vi "Write Bit Field.vi"(5 "occurrence":refnum<k4>, 6 "IL Echo(true)":bool=TRUE, 7 "Close IL Connections (T)":bool=TRUE, 8 "error in (no error)":errorcluster, 9 "Interlock Chain":refnum<class "Interlock Chain.lvclass">, 10 "Bit Field":u16, 11 "Valve in":refnum<class "Valve.lvclass">) -> (0 "error out":errorcluster, 1 "Interlock occured?":bool, 3 "Valve out":refnum<class "Valve.lvclass">)   [LabVIEW 2015, in "cRIO-Carbondioxide.lvlib" / "CO2-Actor.lvlib" / "Valve.lvclass"]
uses:
  Valve.lvclass
  Interlocks/Interlock Chain/Interlock Chain.lvclass
  <vilib>/ActorFramework/Actor/Actor.lvclass/Actor.ctl
  <vilib>/ActorFramework/Message Enqueuer/Message Enqueuer.lvclass/Message Enqueuer.ctl
  Valve.lvclass/Valve.ctl
  <vilib>/ActorFramework/Actor/Read Self Enqueuer.vi
  <vilib>/ActorFramework/Message Enqueuer/Init from Existing Queue.vi
  <vilib>/ActorFramework/Message Enqueuer/Message Enqueuer.lvclass
  <vilib>/ActorFramework/Actor/Actor.lvclass
  CO2 Actor/CO2 Actor.lvclass
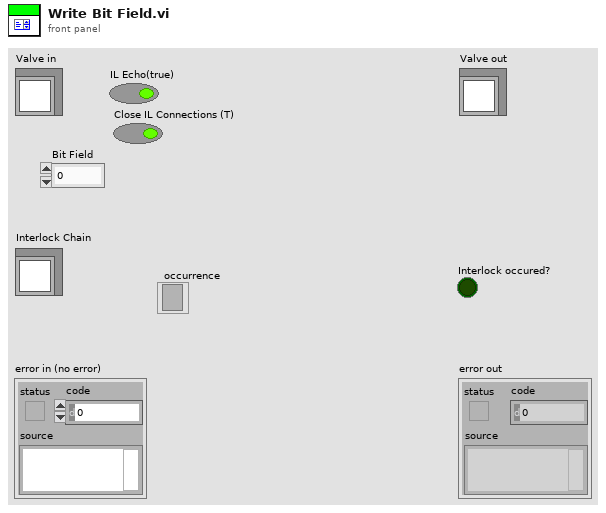
[diagram p1: front panel]
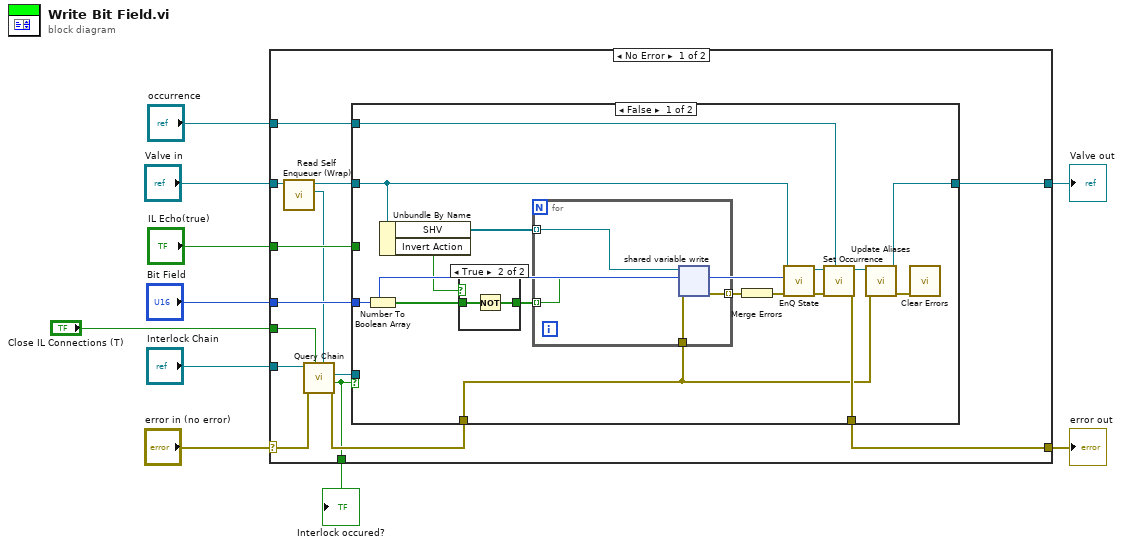
[diagram p0: block diagram]
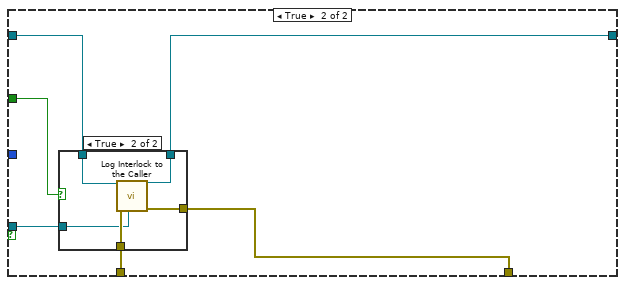
[diagram p3: hidden frame]
diagram:
  n1 = case shown="No Error" "error in (no error)" {
    selector: "error in (no error)" -> [w21 w62]
    tunnel: [w23 w62] -> w9
    tunnel: [w24 w61] -> w7
    tunnel: "Valve in" -> [w13 w61]
    tunnel: "Interlock Chain" -> [w22 _]
    tunnel: "Bit Field" -> [w19 _]
    tunnel: "IL Echo(true)" -> [w17 _]
    tunnel: "Close IL Connections (T)" -> [w16 _]
    tunnel: [w15 _] -> w2
    tunnel: "occurrence" -> [w14 _]
    frame No Error {
      n2 = call "Read Self Enqueuer (Wrap).vi"("CO2 Actor in"=w13) -> ("Actor Framework:Message Enqueuer"=w11:refnum<class "Message Enqueuer.lvclass">, "CO2 Actor out"=w12:refnum<class "Valve.lvclass">)  [unwired: 9 in]
      n3 = call "Query Chain.vi"("Caller Enqueuer"=w11, "Close Connections (F)"=w16, "error in (no error)"=w21, "Interlock Chain"=w22) -> ("error out"=w20:errorcluster, "Interlock?"=w15:bool, "Interlock out"=w18:refnum<class "Interlock.lvclass">)  [unwired: 2 in, 3 out]
      n4 = case shown="False" w15 {
        tunnel: [w34 w50] -> w24
        tunnel: w12 -> [w36 w53]
        tunnel: [w28 w49] -> w23
        tunnel: w20 -> [w25 w52]
        tunnel: w19 -> [w35 _]
        tunnel: w18 -> [_ w51]
        tunnel: w17 -> [_ w48]
        tunnel: w14 -> [w26 _]
        frame False {
          n5 = Number To Boolean Array(number=w35) -> (Boolean array=w39:bool[])
          n6 = Unbundle By Name(w36) -> ("SHV"=w40:refnum<k21>[], "Invert Action"=w31:bool)
          n7 = case shown="True" w31 {
            tunnel: w39 -> [w41 w43]
            tunnel: [w41 w42] -> w32
            frame False {
            }
            frame True {
              n8 = Not(x=w43) -> (.not. x?=w42:bool[])
            }
          }
          n9 = for {
            tunnel: w40 -> [w47] mode=indexing
            tunnel: w32 -> [w45] mode=indexing
            tunnel: w25 -> [w46]
            tunnel: [w44] -> w38 mode=indexing
            n10 = shared-variable-write(w47, w46, w45) -> (w44:errorcluster)  [unwired: 1 out]
          }
          n11 = Merge Errors(w38) -> (w37:errorcluster)
          n12 = call "EnQ State.vi"("error in (no error)"=w37, "BitField"=w35, "Valve in"=w36) -> ("error out"=w29:errorcluster, "Valve out"=w30:refnum<class "Valve.lvclass">)  [unwired: 7 in]
          n13 = call "Set Occurrence.vi"("occurrence"=w26, "error in (no error)"=w29, "Valve in"=w30) -> ("error out"=w28:errorcluster, "Valve out"=w27:refnum<class "Valve.lvclass">)  [unwired: 7 in]
          n14 = call "Update Aliases.vi"("error in (no error)"=w25, "Valve in"=w27) -> ("error out"=w33:errorcluster, "Valve out"=w34:refnum<class "Valve.lvclass">)  [unwired: 8 in]
          n15 = call <vilib>:"Clear Errors.vi"("error in (no error)"=w33) -> ()  [unwired: 5 in, 2 out]
        }
        frame True {
          n16 = case shown="True" w48 {
            tunnel: w53 -> [w54 w57]
            tunnel: w52 -> [w55 w60]
            tunnel: w51 -> [_ w59]
            tunnel: [w54 w56] -> w50
            tunnel: [w55 w58] -> w49
            frame False {
            }
            frame True {
              n17 = call-dynamic "Log Interlock to the Caller.vi"("Interlock in"=w59, "error in (no error)"=w60, "CO2 Actor in"=w57) -> ("error out"=w58:errorcluster, "CO2 Actor out"=w56:refnum<class "Valve.lvclass">)  [unwired: 7 in]
            }
          }
        }
      }
    }
    frame Error {
    }
  }
  "error out" <- w9
  "Valve out" <- w7
  "Interlock occured?" <- w2
